vi "2023-BeginLogic.vi"(1 "error in (no error)":errorcluster) -> (0 "error out":errorcluster)   [LabVIEW 2020]
uses:
  2023 Robot Global Data.vi
panel:
  out "robotID":string="981-2023"
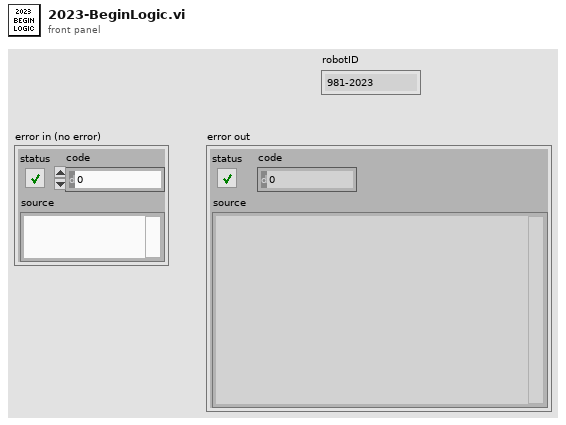
[diagram p1: front panel]
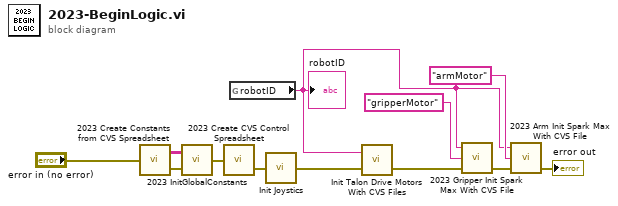
[diagram p0: block diagram]
diagram:
  n1 = call "2023 Create Constants from CVS Spreadsheet.vi"("error in"="error in (no error)") -> ("localConstantSpreadSheet"=w8:string[][], "error out"=w9:errorcluster)
  n2 = call "2023 InitGlobalConstants.vi"("error in (no error)"=w9, "localConstantSpreadSheet"=w8) -> ("error out"=w10:errorcluster)
  n3 = call "2023 Create CVS Control Spreadsheet.vi"("error in"=w10) -> ("error out"=w11:errorcluster)  [unwired: 1 out]
  n4 = global read "2023 Robot Global Data.vi" "robotID"() -> (w3:string)
  "robotID" <- w3
  n5 = call "Init Joystics.vi"("error in"=w11) -> ("error out"=w2:errorcluster)
  n6 = call "Init Talon Drive Motors With CVS Files.vi"("error in"=w2, "Robot ID"=w3) -> ("error out"=w1:errorcluster)  [unwired: 1 out]
  n7 = call "2023 Gripper Init Spark Max With CVS File.vi"("error in"=w1, "Motor ID"="gripperMotor", "Robot ID"=w3) -> ("error out"=w6:errorcluster)  [unwired: 1 in, 1 out]
  n8 = call "2023 Arm Init Spark Max With CVS File.vi"("error in"=w6, "Motor ID"="armMotor", "Robot ID"=w3) -> ("error out"=→"error out":errorcluster)  [unwired: 1 in, 1 out]
